vi "Write Default to File.vi"(8 "error in (no error)":errorcluster, 9 "Name":string, 10 "Path":path, 11 "Rectangle Settings in":refnum<class "Rectangle Settings.lvclass">) -> (0 "error out":errorcluster, 3 "Rectangle Settings out":refnum<class "Rectangle Settings.lvclass">)   [LabVIEW 2019, in "Rectangle Settings.lvclass"]
uses:
  Rectangle Settings.lvclass
  ObjectSettings/ObjectSettings.lvclass
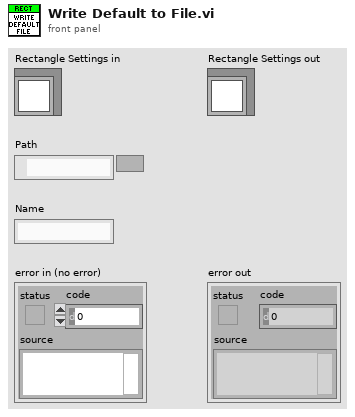
[diagram p1: front panel]
types:
  T1 = typedef "Rectangle Settings.lvclass/Default Rectangle Cluster.ctl" = cluster{"Fill Orientation":u16, "Fill Spacing":dbl}
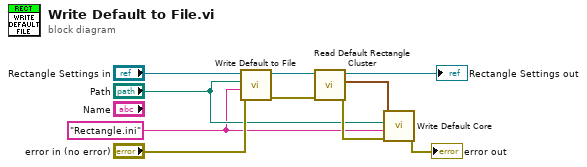
[diagram p0: block diagram]
diagram:
  w2 = "Rectangle.ini"
  n1 = call-parent "Write Default to File.vi"("error in (no error)"="error in (no error)", "Name"=w2, "Path"="Path", "ObjectSettings in"="Rectangle Settings in") -> ("error out"=w6:errorcluster, "ObjectSettings out"=w8:refnum<class "Rectangle Settings.lvclass">)  [unwired: 6 in]
  n2 = call "Read Default Rectangle Cluster.vi"("error in (no error)"=w6, "Rectangle Settings in"=w8) -> ("error out"=w5:errorcluster, "Default Rectangle Cluster"=w4:T1, "Rectangle Settings out"=→"Rectangle Settings out":refnum<class "Rectangle Settings.lvclass">)  [unwired: 7 in]
  n3 = call "Write Default Core.vi"("error in (no error)"=w5, "Name"=w2, "Path"="Path", "Cluster In"=w4) -> ("error out"=→"error out":errorcluster)  [unwired: 6 in, 1 out]
